vi "Dashboard Main.vi"() -> ()   [LabVIEW 2012]
uses:
  DIOOutput.ctl
  SensorsOutput.ctl
  <vilib>/event_ctls.llb/eventvkey.ctl
  <vilib>/Utility/config.llb/Read Key (String).vi
  <vilib>/Utility/config.llb/Read Key (I32).vi
  <vilib>/Utility/config.llb/Write Key (I32).vi
  <vilib>/Utility/config.llb/Write Key (String).vi
  <vilib>/Utility/config.llb/NI_LVConfig.lvlib
panel:
  out "LogFile 2":refnum<file>
  out "LogFile":refnum<file>
  in  "LogString":string
  out "Battery Value":dbl(slide) scale=0.0..14.0 scale format="%#_2e"
  out "Battery":sgl(graph)
  in  "Camera Settings":T1={"Frate Rate"=30, "Compression"=30, "Size"=1} {"Frate Rate" scale=1.0..30.0; "Size" items=["640x480", "320x240", "160x120"]}
  out "Mode":T2(ring)=enum."Auto Disabled"
  out "Camera IP":string
  out "JS1 Z":dbl(slide) scale=-1.0..1.0 scale format="%#_2e"
  out "JS2 Z":dbl(slide) scale=-1.0..1.0 scale format="%#_2e"
  out "Joystick 1":cluster{"X":dbl, "Y":dbl}[](graph)
  out "Joystick 2":cluster{"X":dbl, "Y":dbl}[](graph)
  out "JS Buttons 1":T3
  out "JS Buttons 2":T3
  out "MotorSlide4":dbl(slide) scale=-1.0..1.0 scale format="%#_2e"
  out "MotorSlide3":dbl(slide) scale=-1.0..1.0 scale format="%#_2e"
  out "MotorSlide2":dbl(slide) scale=-1.0..1.0 scale format="%#_2e"
  in  "MotorName3":string="Front Left"
  in  "MotorName4":string="Front Right"
  in  "MotorName1":string="Rear Left"
  in  "MotorName2":string="Rear Right"
  out "MotorChart4":dbl(graph)
  out "MotorChart3":dbl(graph)
  out "MotorChart2":dbl(graph)
  out "MotorSlide1":dbl(slide) scale=-1.0..1.0 scale format="%#_2e"
  out "MotorChart1":dbl(graph)
  out "Robot IP":string
  in  "Dashboard Tab":T4(tab)
  in  "Single Stick":bool
  in  "Shooter Scale":dbl(knob)=0.7000000000000001 min=0.1 max=1.0 step=0.1 scale=0.1..1.0 scale format="%#.1g"
  in  "Tank_Drive":bool
  out "DIO Template":T5
  out "Sensors":T6
  out "Target Info":T7(array[cluster])
  in  "Slider":dbl(slide) scale=0.0..100.0 scale format="%#_3g"
  in  "On/Off":bool caption="Solenoid"
  in  "Test Name":u16(ring) items=["Select the test to run...", "Example Test", "-------------------------------", "List of tests is built in robot code.", "Replace with your own automated tests."]
  in  "Test Tree":string(tree)
  in  "Motor":cluster{"Value":dbl, "Enable":bool} {"Value" scale=-1.0..1.0 scale format="%#_3g"}
  out "Progress":T8 {"Test Progress" scale=0.0..100.0}
  in  "Rev/Fwd":cluster{"Forward":bool, "Reverse":bool}
  in  "Ring":u16(ring) items=["Auto", "Fixed indoor", "Fixed outdoor 1", "Fixed outdoor 2", "Fixed fluorescent 1", "Fixed fluorescent 2", "Hold current"]
  in  "Listbox":i32(listbox)
  in  "Viewer":T9(tab)
  out "Mbps":dbl format="%#.1g"
  in  "Enable":bool
  in  "DB Camera Config":bool
  out "Mbps":bool
  out "fps":dbl format="%#.1g"
  out "Image Error Message":string="Timeout in Camera Communications"
  out "Camera Image":T10(plugin-control)
  out "Buttons 1":cluster{"1":bool, "2":bool, "3":bool}
  out "Kinect 1":cluster{"X":dbl, "Y":dbl, "Z":dbl} {"X" scale=1.0..-1.0; "Y" scale=1.0..-1.0; "Z" scale=1.0..-1.0}
  out "Buttons 2":cluster{"1":bool, "2":bool, "3":bool}
  out "Kinect 2":cluster{"X":dbl, "Y":dbl, "Z":dbl} {"X" scale=1.0..-1.0; "Y" scale=1.0..-1.0; "Z" scale=1.0..-1.0}
  out "Version":string
  out "Skeleton Picture":picture
  out "Players":i8
  out "Tree":string(tree)
  # "Drive & Motors"
  # "Robot IP:"
  # "Arcade Drive"
  # "Tank Drive"
  # "Double Stick"
  # "Single Stick"
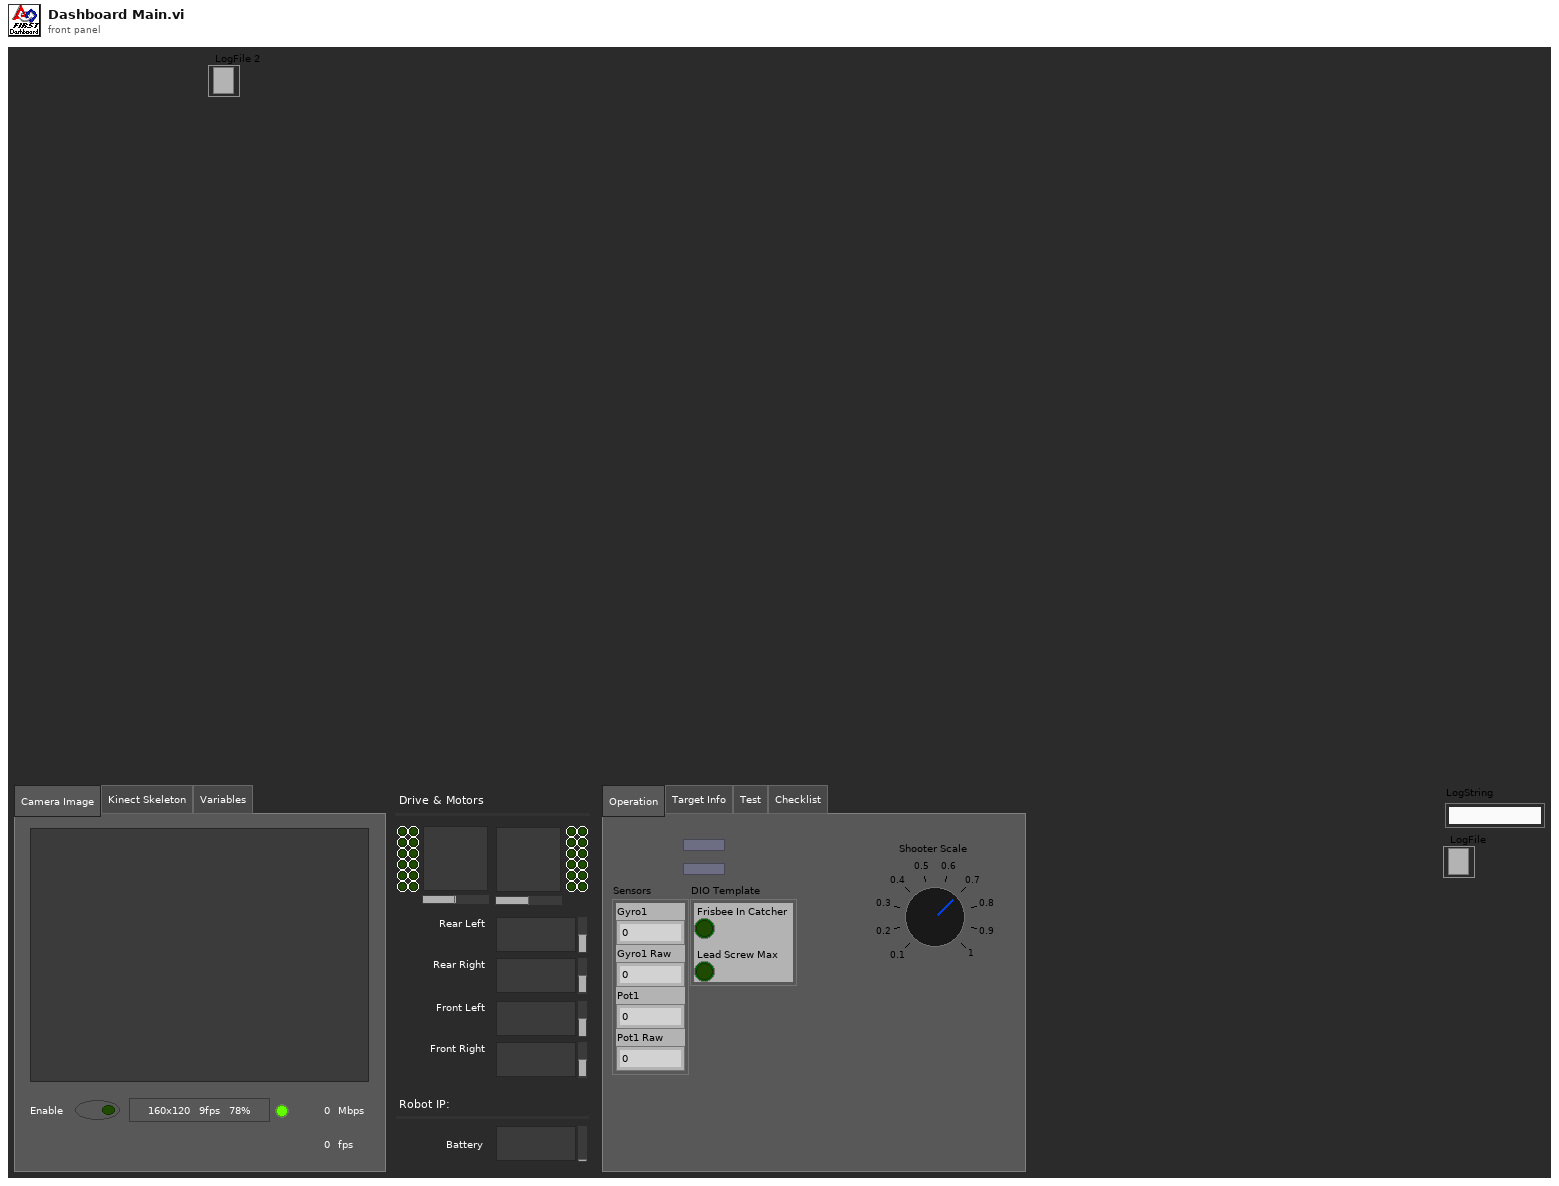
[diagram p1: front panel]
types:
  T1 = cluster{"Frate Rate":i32, "Compression":i32, "Size":u16}
  T2 = enum8{"Tele-Op Disabled", "Tele-Op Enabled", "Auto Disabled", "Auto Enabled", "Test Disabled", "Test Enabled", ""}
  T3 = cluster{bool, bool, bool, bool, bool, bool, bool, bool, bool, bool, bool, bool}
  T4 = enum32{"Operation", "Target Info", "Test", "Checklist"}
  T5 = typedef "DIOOutput.ctl" = cluster{"Frisbee In Catcher":bool, "Lead Screw Max":bool}
  T6 = typedef "SensorsOutput.ctl" = cluster{"Gyro1":dbl, "Gyro1 Raw":dbl, "Pot1":dbl, "Pot1 Raw":dbl}
  T7 = cluster{"Center Position":cluster{"X":dbl, "Y":dbl}, "Distance (ft)":dbl, "Center":bool}[]
  T8 = cluster{"Test Progress":u8, "Test Progress Text":string}
  T9 = enum32{"Camera Image", "Kinect Skeleton", "Variables"}
  T10 = typedef "IMAQ Image.ctl" = refnum<image>
  T11 = enum16{"open", "replace", "create", "open or create", "replace or create", "replace or create with confirmation"}
  T12 = typedef "Image Type" = u32
  T13 = typedef "LVBoundsTypeDef.ctl" = cluster{"Width":u32, "Height":u32}
  T14 = typedef "SkeletonTrackState.ctl" = enum32{"NotTracked", "PositionOnly", "Tracked"}
  T15 = cluster{"TrackingState":u8[], "Position":cluster{"x":sgl, "y":sgl, "z":sgl}, cluster{"x":sgl, "y":sgl, "z":sgl, sgl}[], "TrackState":T14}
  T16 = cluster{cluster{"ScaledToPercentRange":dbl, "ScaledToPercentRange":dbl, "ScaledToPercentRange":dbl}, cluster{bool, bool, bool}}[]
  T17 = cluster{cluster{"ScaledToPercentRange":dbl, "ScaledToPercentRange":dbl, "ScaledToPercentRange":dbl}, cluster{bool, bool, bool}}
  T18 = cluster{"ScaledToPercentRange":dbl, "ScaledToPercentRange":dbl, "ScaledToPercentRange":dbl}
  T19 = typedef "LVRectTypeDef.ctl" = cluster{"Left":i16, "Top":i16, "Right":i16, "Bottom":i16}
  T20 = cluster{"Competition mode":bool, "Robot Link":bool, "Autonomous":bool, "Enabled":bool, "E-Stop":bool, "Simulated":bool, "TestMode":bool, "Docked Window":bool}
  T21 = cluster{"Boolean Array[0]":bool, "Boolean Array[1]":bool, "Boolean Array[2]":bool, "Boolean Array[3]":bool, "Boolean Array[4]":bool, "Boolean Array[5]":bool, "Boolean Array[6]":bool, "Boolean Array[7]":bool, "Boolean Array[8]":bool, "Boolean Array[9]":bool, "Boolean Array[10]":bool, "Boolean Array[11]":bool}
  T22 = cluster{"Position":cluster{"X":dbl, "Y":dbl}, "Distance (ft)":dbl, "Center":bool}[]
  T23 = cluster{cluster{"Numeric":dbl, "Numeric":dbl}, "Numeric":dbl, bool}
  T24 = cluster{"Position":cluster{"Numeric":dbl, "Numeric":dbl}, "Numeric":dbl, "Center":bool}[]
  T25 = typedef "NI_LVConfig.lvlib/Config Data RefNum.ctl" = refnum<k1>
  T26 = typedef "LVDateTimeRec.ctl" = cluster{"fractional second":dbl, "second":i32, "minute":i32, "hour":i32, "day of month":i32, "month":i32, "year":i32, "day of week":i32, "day of year":i32, "DST":i32}
  T27 = typedef "eventvkey.ctl" = enum16{"ASCII", "Enter", "Return", "Shift", "Ctrl", "Alt", "Cmd", "Opt", "Caps", "NumLock", "Clear", "Break", "Up", "Down", "Left", "Right", "Insert", "Delete", "Home", "End", "PageUp", "PageDown", "Escape", "Help", "Pause", "ScrollLock", "F1", "F2", "F3", "F4", "F5", "F6", "F7", "F8", "F9", "F10", "F11", "F12", "F13", "F14", "F15", "F16", "F17", "F18", "F19", "F20", "F21", "F22", "F23", "F24", "Play", "VolumeUp", "VolumeDown", "Mute", "Two Byte Char"}
  T28 = cluster{"Numeric Array[0]":dbl, "Numeric Array[1]":dbl, "Numeric Array[2]":dbl, "Numeric Array[3]":dbl, "Numeric Array[4]":dbl, "Numeric Array[5]":dbl, "Numeric Array[6]":dbl, "Numeric Array[7]":dbl, "Numeric Array[8]":dbl}
  T29 = cluster{"Boolean Array[0]":bool, "Boolean Array[1]":bool, "Boolean Array[2]":bool, "Boolean Array[3]":bool, "Boolean Array[4]":bool, "Boolean Array[5]":bool, "Boolean Array[6]":bool, "Boolean Array[7]":bool, "Boolean Array[8]":bool}
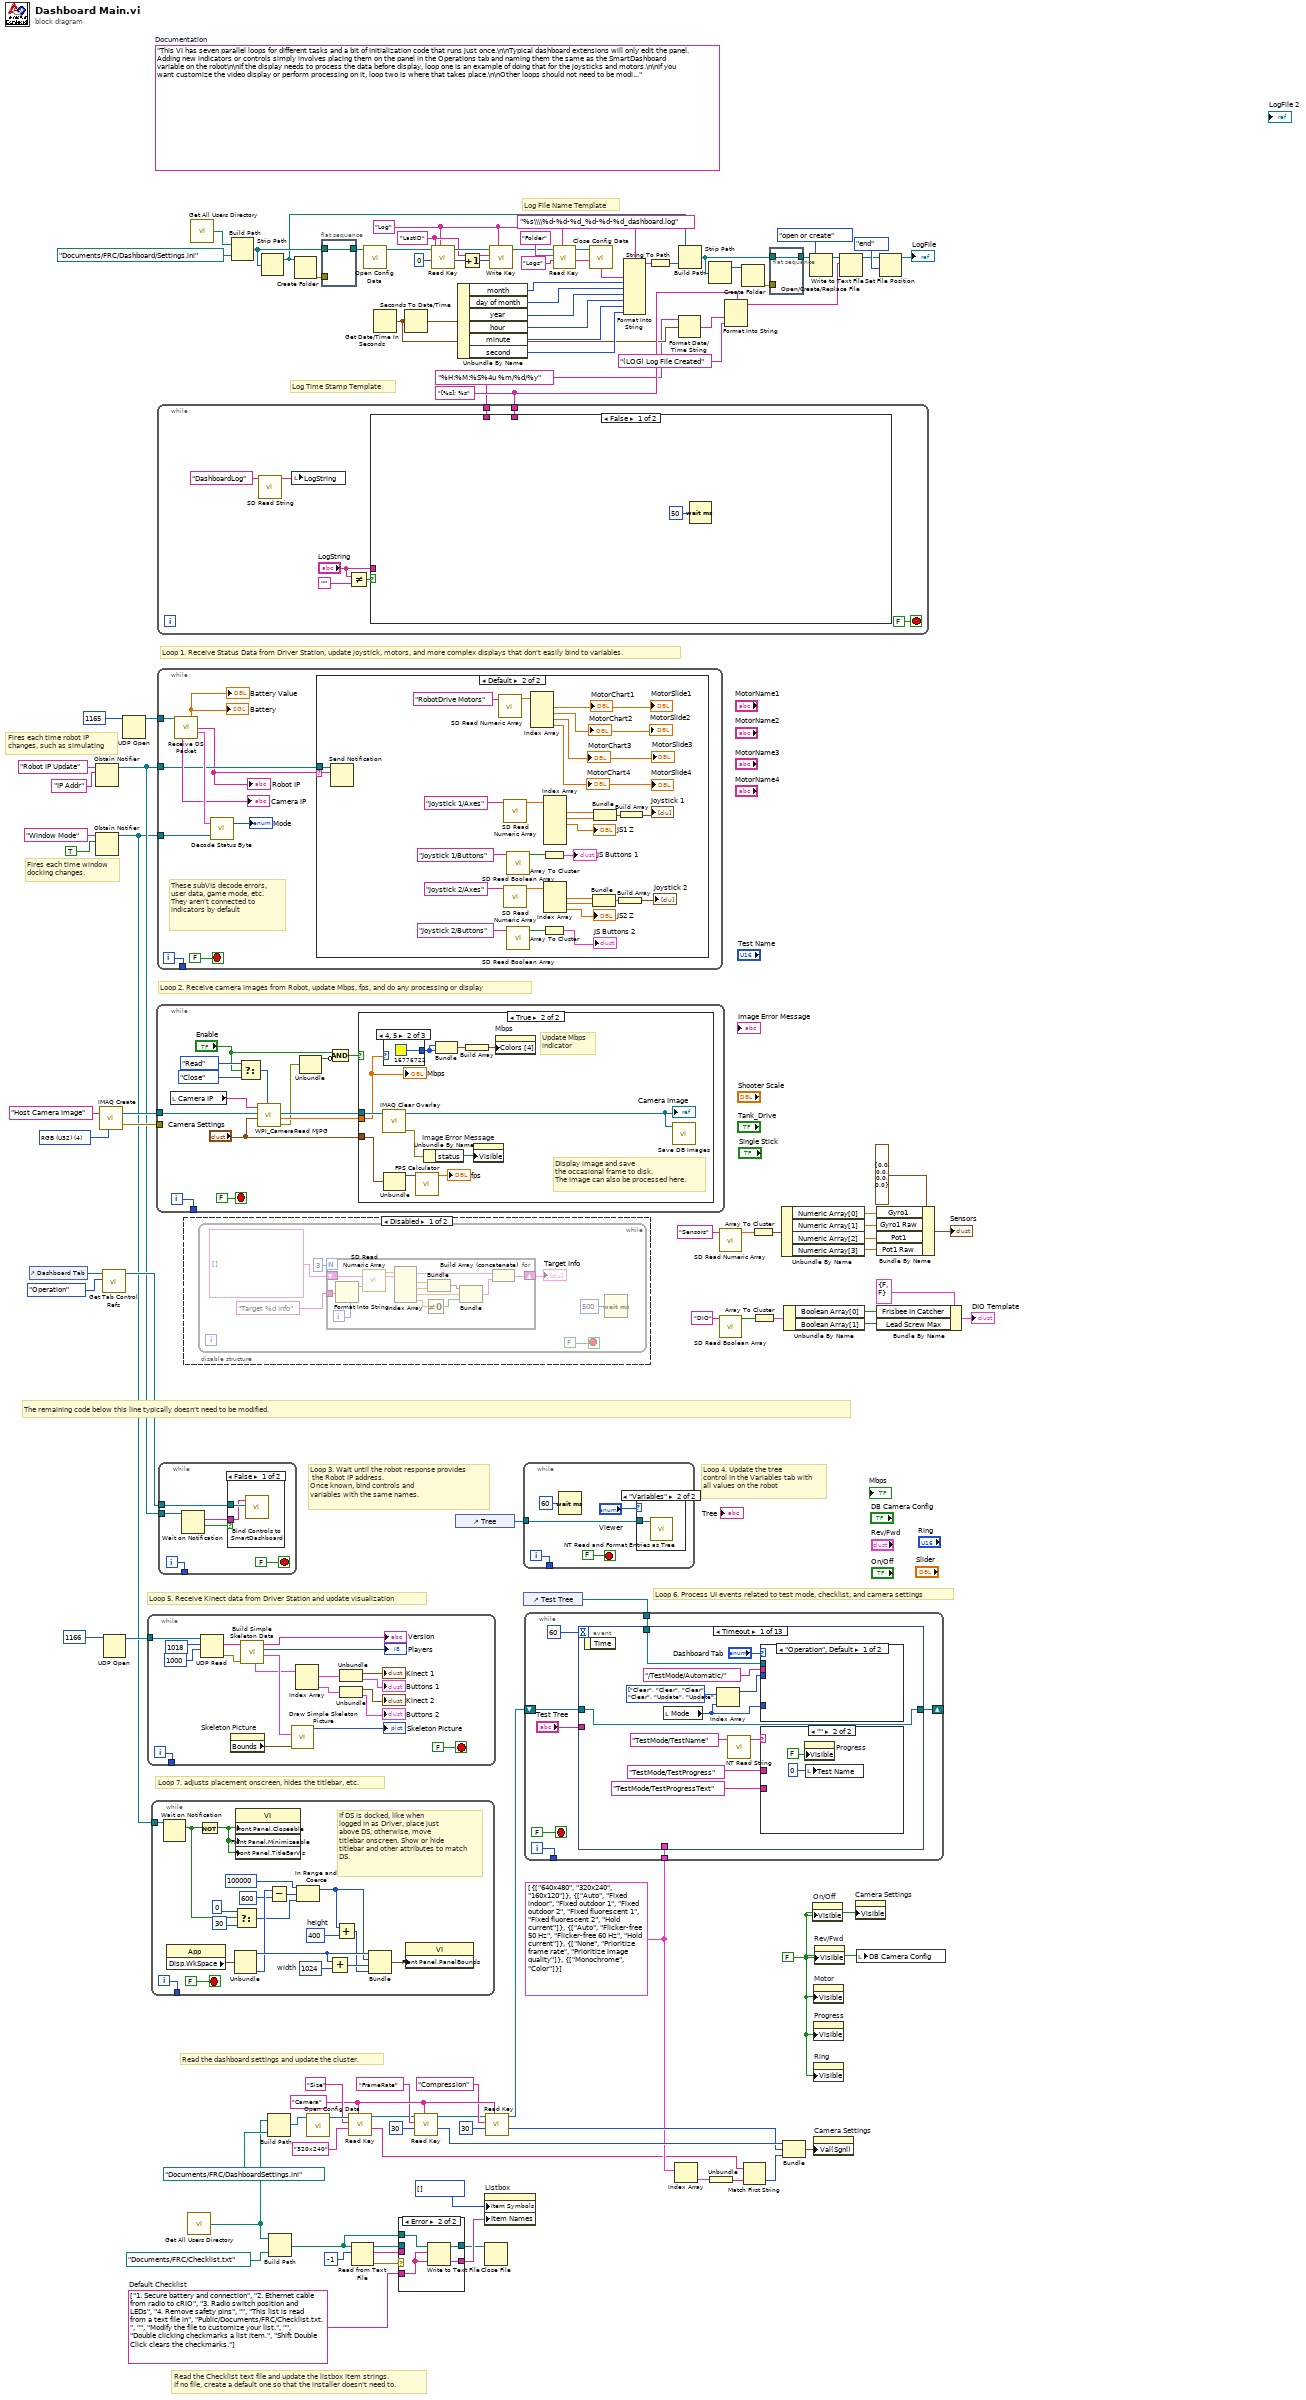
[diagram p0: block diagram]
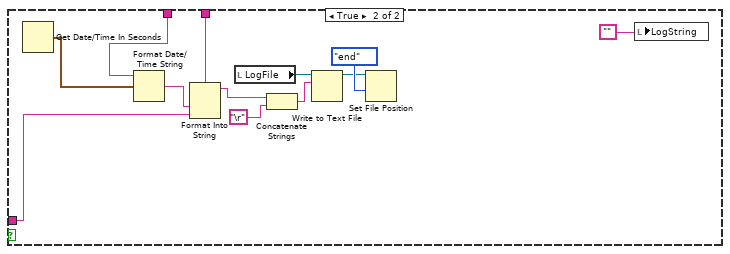
[diagram p2: hidden frame]
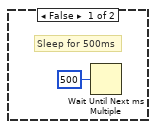
[diagram p5: hidden frame]
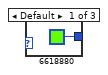
[diagram p6: hidden frame]
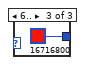
[diagram p7: hidden frame]
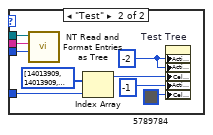
[diagram p9: hidden frame]
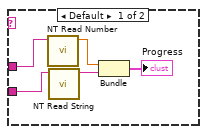
[diagram p10: hidden frame]
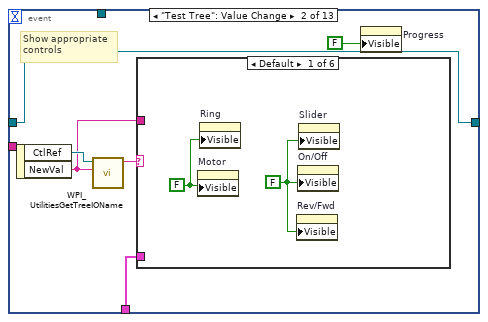
[diagram p11: hidden frame]
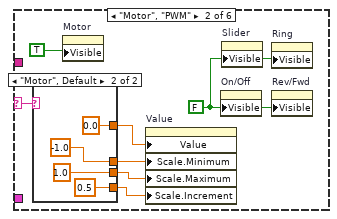
[diagram p12: hidden frame]
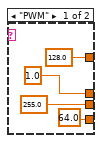
[diagram p13: hidden frame]
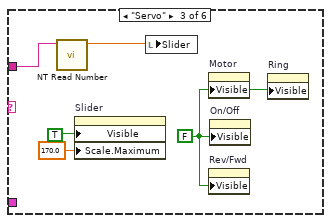
[diagram p14: hidden frame]
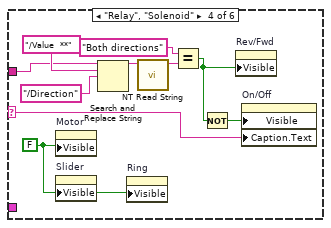
[diagram p15: hidden frame]
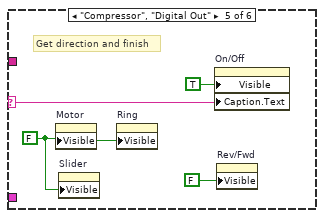
[diagram p16: hidden frame]
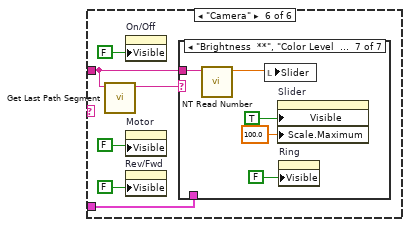
[diagram p17: hidden frame]
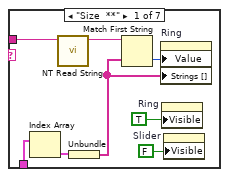
[diagram p18: hidden frame]
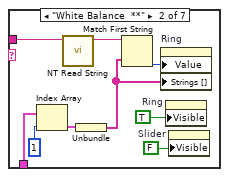
[diagram p19: hidden frame]
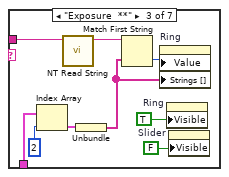
[diagram p20: hidden frame]
diagram:
  w17 = "%H:%M:%S%4u %m/%d/%y"
  w23 = "[%s]: %s"
  w50 = "LastID" ("key")
  w49 = "Log" ("section")
  w81 = "Camera"
  w73 = cluster{string[]}[] [{["640x480", "320x240", "160x120"]}, {["Auto", "Fixed indoor", "Fixed outdoor 1", "Fixed outdoor 2", "Fixed fluorescent 1", "Fixed fluorescent 2", "Hold current"]}, {["Auto", "Flicker-free 50 Hz", "Flicker-free 60 Hz", "Hold current"]}, {["None", "Prioritize frame rate", "Prioritize image quality"]}, {["Monochrome", "Color"]}]
  w88 = string[] ["1. Secure battery and connection", "2. Ethernet cable from radio to cRIO", "3. Radio switch position and LEDs", "4. Remove safety pins", "", "This list is read from a text file in", "Public/Documents/FRC/Checklist.txt.", "", "Modify the file to customize your list.", "", "Double clicking checkmarks a list item.", "Shift Double Click clears the checkmarks."]  # Default Checklist
  w86 = FALSE ("Visible")
  (unwired) "This VI has seven parallel loops for different tasks and a bit of initialization code that runs just once.\n\nTypical dashboard extensions will only edit the panel. Adding new indicators or controls simply involves placing them on the panel in the Operations tab and naming them the same as the SmartDashboard variable on the robot\n\nIf the display needs to process the data before display, loop one is an example of doing that for the joysticks and motors.\n\nIf you want customize the video display or perform processing on it, loop two is where that takes place.\n\nOther loops should not need to be modified. They are pretty standard, and document the task they perform."  # Documentation
  w109 = T12 4 items=["Grayscale (U8)", "Grayscale (I16)", "Grayscale (SGL)", "Complex (CSG)", "RGB (U32)", "HSL (U32)", "RGB (U64)"] ("Image Type")
  # "Log File Name Template"
  # "Log Time Stamp Template"
  # "Fires each time robot IP\nchanges, such as simulating"
  # "Fires each time window\ndocking changes."
  # "Read the Checklist text file and update the listbox item strings.\nIf no file, create a default one so that the installer doesn't need to."
  # "The remaining code below this line typically doesn't need to be modified."
  # "Loop 6. Process UI events related to test mode, checklist, and camera settings"
  # "Read the dashboard settings and update the cluster."
  # "Loop 4. Update the tree\ncontrol in the Variables tab with\nall values on the robot"
  # "Loop 3. Wait until the robot response provides\n the Robot IP address.\nOnce known, bind controls and\nvariables with the same names."
  # "Loop 5. Receive Kinect data from Driver Station and update visualization"
  # "Loop 7. adjusts placement onscreen, hides the titlebar, etc."
  # "Loop 1. Receive Status Data from Driver Station, update joystick, motors, and more complex displays that don't easily bind to variables."
  # "Loop 2. Receive camera images from Robot, update Mbps, fps, and do any processing or display"
  n1 = control-ref of="Dashboard Tab"() -> (w102:refnum<vi>)
  n2 = Obtain Notifier(name (unnamed)="Robot IP Update", notification data type="IP Addr" ("name (unnamed)")) -> (notifier out=w99:refnum<notifier>)  [unwired: 2 in, 2 out]
  n3 = Obtain Notifier(name (unnamed)="Window Mode", notification data type=TRUE) -> (notifier out=w92:refnum<notifier>)  [unwired: 2 in, 2 out]
  n4 = call "IMAQ Create"("Image Name"="Host Camera Image", "Image Type"=w109) -> ("New Image"=w107:T10, "error out"=w106:errorcluster)  [unwired: 2 in, 1 out]
  n5 = call <vilib>:"Get Tab Control Refs.vi"("Page Index"=enum32{"Operation", "Test"}."Operation" ("Dashboard Tab"), "TabControl in"=w102) -> ("ControlsOnPage"=w103:refnum<vi>[])  [unwired: 9 in]
  n6 = UDP Open(11:u16 1166 ("port")) -> (port=w104:refnum<k16>)  [unwired: 2 in, 4 out]
  n7 = UDP Open(11:u16 1165 ("port")) -> (port=w110:refnum<k16>)  [unwired: 2 in, 4 out]
  n8 = while {
    tunnel: w104 -> [w128]
    tunnel: [w113] -> _
    i -> [w113]
    stop <- FALSE stop-if-true
    n9 = UDP Read(connection ID=w128, max size (548)=1018 ("bytes to read"), timeout ms (25000)=1000) -> (data out=w122:string, error out=w112:errorcluster)  [unwired: 1 in, 3 out]
    n10 = property on="Skeleton Picture" class="Pict"() -> ("Bounds"=w124:T13)  [unwired: 2 in, 2 out]
    n11 = call "Build Simple Skeleton Data.vi"("error in (no error)"=w112, "data in"=w122) -> ("Skeleton Data"=w123:T15, "NumPlayers"=→"Players":i8, "Version String"=→"Version":string, "Simple Joystick Info"=w120:T16)  [unwired: 5 in, 1 out]
    n12 = call "Draw Simple Skeleton Picture.vi"("Bounds"=w124, "Simple Skeleton"=w123) -> ("new picture out"=→"Skeleton Picture":picture)  [unwired: 9 in]
    n13 = Index Array(array=w120) -> (element #1=w119:T17, element #2=w118:T17)  [unwired: 2 in]
    n14 = Unbundle(w119) -> (→"Kinect 1":T18, →"Buttons 1":cluster{bool, bool, bool})
    n15 = Unbundle(w118) -> (→"Kinect 2":T18, →"Buttons 2":cluster{bool, bool, bool})
  }
  n16 = while {
    tunnel: w92 -> [w149]
    tunnel: [w147] -> _
    i -> [w147]
    stop <- FALSE stop-if-true
    w139 = 1024  # width
    w142 = 400  # height
    # "If DS is docked, like when\nlogged in as Driver, place just\nabove DS, otherwise, move\ntitlebar onscreen. Show or hide\ntitlebar and other attributes to match\nDS."
    n17 = Wait on Notification(notifier=w149) -> (notification=w134:bool)  [unwired: 3 in, 3 out]
    n18 = property class="App"() -> ("Disp.WkSpace"=w145:T19)  [unwired: 2 in, 2 out]
    n19 = Not(x=w134) -> (.not. x?=w148:bool)
    n20 = Unbundle(w145) -> ("Left"=w143:i16, "Bottom"=w140:i16)  [unwired: 2 out]
    n21 = Select(t=0, s=w134, f=30) -> (s? t:f=w133:i32)
    n22 = property class="VI"("Front Panel.Closeable"=w148, "Front Panel.Minimizeable"=w148, "Front Panel.TitleBarVis"=w148) -> ()  [unwired: 2 in, 2 out]
    n23 = Subtract(x=w140, y=600) -> (x-y=w137:i32)
    n24 = In Range and Coerce(upper limit=100000, x=w137, lower limit=w133) -> (coerced(x)=w131:i32)  [unwired: 1 out]
    n25 = Add(x=w143, y=w139) -> (x+y=w144:i32)
    n26 = Add(x=w131, y=w142) -> (x+y=w141:i32)
    n27 = Bundle("Left"=w143, w131, w144, w141) -> (w146:cluster{"Left":i16, i32, i32, i32})  [unwired: 1 out]
    n28 = property class="VI"("Front Panel.PanelBounds"=w146) -> ()  [unwired: 2 in, 2 out]
  }
  n29 = while {
    tunnel: w107 -> [w160]
    tunnel: w106 -> [_]
    tunnel: [w163] -> _
    i -> [w163]
    stop <- FALSE stop-if-true
    n30 = local read "Camera IP"() -> (w162:string)
    n31 = Select(t=enum16{"Read", "Reopen", "Close"}."Read" ("Operation"), s="Enable", f=enum16{"Read", "Reopen", "Close"}."Close" ("Operation")) -> (s? t:f=w155:enum16{"Read", "Reopen", "Close"})
    n32 = call <vilib>:"WPI_CameraRead MJPG.vi"("Operation"=w155, "Camera Settings"="Camera Settings", "Image"=w160, "address"=w162) -> ("error out"=w154:errorcluster, "Bandwidth (kbps)"=w158:dbl, "Image Out"=w159:T10)  [unwired: 5 in]
    n33 = Unbundle(w154) -> ("status"=w152:bool)  [unwired: 2 out]
    n34 = Compound Arithmetic op=AND("Enable", invert w152) -> (w151:bool)
    n35 = case shown="True" w151 {
      tunnel: "Camera Settings" -> [_ w167]
      tunnel: w159 -> [_ w170]
      tunnel: w158 -> [_ w169]
      frame False {
        # "Sleep for 500ms"
        n36 = Wait Until Next ms Multiple(millisecond multiple=u32 500) -> ()  [unwired: 1 out]
      }
      frame True {
        # "Display image and save\nthe occasional frame to disk.\nThe image can also be processed here."
        # "Update Mbps\nindicator"
        n37 = call "IMAQ Clear Overlay"("Image"=w170) -> ("error out"=w175:errorcluster, "Image Out"=w174:T10)  [unwired: 2 in, 7 out]
        "Camera Image" <- w174
        n38 = case shown="4, 5" w169 {
          tunnel: [u32 6618880 ("Color Box") u32 16776722 ("Color Box") u32 16716800 ("Color Box")] -> w171
          frame Default {
          }
          frame 4, 5 {
          }
          frame 6.. {
          }
        }
        n39 = Unbundle(w167) -> ("Frate Rate"=w166:i32)  [unwired: 2 out]
        n40 = call "FPS Calculator.vi"("Average Count"=w166) -> ("fps"=→"fps":dbl)  [unwired: 10 in]
        n41 = Unbundle By Name(w175) -> ("status"=w176:bool)
        n42 = Bundle("Color Box"=w171, "Color Box"=w171) -> (w173:cluster{"Color Box":u32, "Color Box":u32})  [unwired: 1 out]
        n43 = Build Array(w173) -> (w172:cluster{"Color Box":u32, "Color Box":u32}[])
        n44 = property on="Image Error Message" class="Str"("Visible"=w176) -> ()  [unwired: 2 in, 2 out]
        n45 = property on="Mbps" class="Bool (strict)"("Colors [4]"=w172) -> ()  [unwired: 2 in, 2 out]
        n46 = call "Save DB Images.vi"("Image"=w174) -> ()  [unwired: 2 in, 1 out]
        "Mbps" <- w169
      }
    }
  }
  n47 = while {
    tunnel: w23 -> [w184]
    tunnel: w17 -> [w182]
    stop <- FALSE stop-if-true
    n48 = call <vilib>:"SD Read String.vi"("Name"="DashboardLog") -> ("String"=w180:string)  [unwired: 8 in, 2 out]
    n49 = local write "LogString"(w180) -> ()
    n50 = Not Equal?(x="LogString", y="") -> (x != y?=w186:bool)
    n51 = case shown="False" w186 {
      tunnel: "LogString" -> [_ w189]
      tunnel: w184 -> [_ w197]
      tunnel: w182 -> [_ w191]
      frame False {
        n52 = Wait (ms)(milliseconds to wait=u32 50) -> ()  [unwired: 1 out]
      }
      frame True {
        n53 = Get Date/Time In Seconds() -> (seconds since 1Jan1904=w192:timestamp)
        n54 = Format Date/Time String(time format string (%c)=w191, seconds (now)=w192) -> (date/time string=w190:string)  [unwired: 1 in]
        n55 = Format Into String(format string=w197, w190, w189) -> (resulting string=w194:string)  [unwired: 2 in, 1 out]
        n56 = local read "LogFile"() -> (w198:refnum<file>)
        n57 = Concatenate Strings(w194, "\r") -> (w195:string)
        n58 = Write to Text File(file (use dialog)=w198, text=w195) -> (refnum out=w199:refnum<file>)  [unwired: 2 in, 2 out]
        n59 = Set File Position(refnum=w199, from (0:start)=enum16{"start", "end", "current"}."end") -> ()  [unwired: 2 in, 2 out]
        n60 = local write "LogString"("") -> ()
      }
    }
  }
  n61 = while {
    tunnel: w110 -> [w208]
    tunnel: w99 -> [w202]
    tunnel: w92 -> [w206]
    tunnel: [w203] -> _
    i -> [w203]
    stop <- FALSE stop-if-true
    # "These subVIs decode errors, user data, game mode, etc.\nThey aren't connected to indicators by default"
    n62 = call "Receive DS Packet.vi"("Recv Socket"=w208) -> ("Battery"=→"Battery" →"Battery Value":sgl, "Robot IP Address"=w201:string, "Status"=w209:T20, "Camera IP Address"=→"Camera IP":string)  [unwired: 1 in, 10 out]
    "Robot IP" <- w201
    n63 = call "Decode Status Byte.vi"("Window Mode Notifier"=w206, "Status"=w209) -> ("Mode"=→"Mode":T2)  [unwired: 1 out]
    n64 = case shown="Default" w201 {
      selector: w201 -> [_ w211]
      tunnel: w202 -> [_ w212]
      frame "0.0.0.0" {
        # "Robot not responding, don't poll the variables"
      }
      frame Default {
        n65 = Send Notification(notification=w211, notifier=w212) -> ()  [unwired: 1 in, 2 out]
        n66 = call <vilib>:"SD Read Numeric Array.vi"("Name"="RobotDrive Motors") -> ("Numeric Array"=w235:dbl[])  [unwired: 8 in, 2 out]
        n67 = call <vilib>:"SD Read Numeric Array.vi"("Name"="Joystick 1/Axes") -> ("Numeric Array"=w228:dbl[])  [unwired: 8 in, 2 out]
        n68 = call <vilib>:"SD Read Numeric Array.vi"("Name"="Joystick 2/Axes") -> ("Numeric Array"=w222:dbl[])  [unwired: 8 in, 2 out]
        n69 = call <vilib>:"SD Read Boolean Array.vi"("Name"="Joystick 1/Buttons") -> ("Boolean Array"=w230:bool[])  [unwired: 8 in, 2 out]
        n70 = call <vilib>:"SD Read Boolean Array.vi"("Name"="Joystick 2/Buttons") -> ("Boolean Array"=w221:bool[])  [unwired: 8 in, 2 out]
        n71 = Index Array(array=w235) -> (element #1=→"MotorChart1" →"MotorSlide1":dbl, element #2=→"MotorSlide2" →"MotorChart2":dbl, element #3=→"MotorChart3" →"MotorSlide3":dbl, element #4=→"MotorChart4" →"MotorSlide4":dbl)  [unwired: 4 in]
        n72 = Array To Cluster(array=w230) -> (cluster=→"JS Buttons 1":T21)
        n73 = Array To Cluster(array=w221) -> (cluster=→"JS Buttons 2":T21)
        n74 = Index Array(array=w228) -> (element #1=w225:dbl, element #2=w226:dbl, element #3=→"JS1 Z":dbl)  [unwired: 6 in, 3 out]
        n75 = Index Array(array=w222) -> (element #1=w217:dbl, element #2=w216:dbl, element #3=→"JS2 Z":dbl)  [unwired: 3 in]
        n76 = Bundle("Numeric"=w217, "Numeric"=w216) -> (w218:cluster{"Numeric":dbl, "Numeric":dbl})  [unwired: 1 in]
        n77 = Bundle("Numeric"=w225, "Numeric"=w226) -> (w224:cluster{"Numeric":dbl, "Numeric":dbl})  [unwired: 1 in]
        n78 = Build Array(w218) -> (→"Joystick 2":cluster{"Numeric":dbl, "Numeric":dbl}[])
        n79 = Build Array(w224) -> (→"Joystick 1":cluster{"Numeric":dbl, "Numeric":dbl}[])
      }
    }
  }
  n80 = while {
    tunnel: w103 -> [w244]
    tunnel: w99 -> [w241]
    tunnel: [w239] -> _
    i -> [w239]
    stop <- FALSE stop-if-true
    n81 = Wait on Notification(notifier=w241) -> (notification=w240:string, timed out?=w242:bool)  [unwired: 3 in, 2 out]
    n82 = case shown="False" w242 {
      tunnel: w244 -> [w246 _]
      tunnel: w240 -> [w245 _]
      frame False {
        n83 = call <vilib>:"Bind Controls to SmartDashboard.vi"("Bound Control Refs"=w246, "Server IP Address"=w245) -> ()  [unwired: 10 in]
      }
      frame True {
      }
    }
  }
  n84 = disable-structure shown="Disabled" {
    frame Disabled {
      n85 = while {
        stop <- FALSE stop-if-true
        n86 = for {
          N: 3 -> [_]
          tunnel: "Target %d Info" ("format string") -> [w265]
          shift-right: [w253] -> w249
          shift-left: T22 [] -> [w254]
          i -> [w264]
          n87 = Format Into String(format string=w265, w264) -> (resulting string=w263:string)  [unwired: 2 in, 1 out]
          n88 = call <vilib>:"SD Read Numeric Array.vi"("Name"=w263) -> ("Numeric Array"=w262:dbl[])  [unwired: 8 in, 2 out]
          n89 = Index Array(array=w262) -> (element #1=w256:dbl, element #2=w257:dbl, element #3=w258:dbl, element #4=w261:dbl)  [unwired: 4 in]
          n90 = Not Equal To 0?(x=w261) -> (x != 0?=w260:bool)
          n91 = Bundle("Numeric"=w256, "Numeric"=w257) -> (w259:cluster{"Numeric":dbl, "Numeric":dbl})  [unwired: 1 in]
          n92 = Bundle(w259, "Numeric"=w258, w260) -> (w255:T23)  [unwired: 1 in]
          n93 = Build Array (concatenate)(w254, w255) -> (w253:T24)
        }
        "Target Info" <- w249
        n94 = Wait (ms)(milliseconds to wait=u32 500) -> ()  [unwired: 1 out]
      }
    }
    frame Enabled {
    }
  }
  n95 = call "Get All Users Directory.vi"() -> ("All User Path"=w46:path)
  n96 = call "Get All Users Directory.vi"() -> ("All User Path"=w38:path)
  n97 = Build Path(base path=w38, name or relative path=path "Documents/FRC/Dashboard/Settings.ini") -> (appended path=w43:path)
  n98 = Strip Path(path=w43) -> (stripped path=w35:path)  [unwired: 1 out]
  n99 = Build Path(base path=w46, name or relative path=path "Documents/FRC/DashboardSettings.ini") -> (appended path=w85:path)
  n100 = Build Path(base path=w46, name or relative path=path "Documents/FRC/Checklist.txt") -> (appended path=w89:path)
  n101 = Create Folder(path (use dialog)=w35) -> (error out=w44:errorcluster)  [unwired: 2 in, 2 out]
  n102 = call <vilib>:"Open Config Data.vi"("configuration file path"=w85) -> ("refnum"=w84:T25)  [unwired: 8 in, 2 out]
  n103 = flat-sequence {
    tunnel: w44 -> [_]
    tunnel: [w266] -> w42
    tunnel: w43 -> [w266]
    frame #0 {
    }
  }
  n104 = call-poly <vilib>:"Read Key.vi"("section"=w81, "default value"="320x240", "key"="Size", "refnum"=w84) -> ("value"=w71:string, "refnum out"=w66:T25)  [unwired: 2 in, 4 out]
  n105 = Read from Text File(file (use dialog)=w89, count=-1 ("timeout ms (25000)")) -> (refnum out=w68:refnum<file>, text=w90:string[], error out=w91:errorcluster)  [unwired: 2 in, 1 out]
  n106 = call <vilib>:"Open Config Data.vi"("configuration file path"=w42) -> ("refnum"=w59:T25)  [unwired: 8 in, 2 out]
  n107 = Get Date/Time In Seconds() -> (seconds since 1Jan1904=w18:timestamp)
  n108 = case shown="Error" w91 {
    tunnel: w90 -> [w268 _]
    tunnel: [w268 w270] -> w87
    tunnel: w88 -> [_ w270]
    tunnel: w89 -> [_ w271]
    tunnel: [w267 w269] -> w67
    tunnel: w68 -> [w267 _]
    frame No Error {
    }
    frame Error {
      n109 = Write to Text File(file (use dialog)=w271, text=w270) -> (refnum out=w269:refnum<file>)  [unwired: 2 in, 2 out]
    }
  }
  n110 = Seconds To Date/Time(time stamp (now)=w18) -> (date time rec=w33:T26)  [unwired: 1 in]
  n111 = call-poly <vilib>:"Read Key.vi"("section"=w81, "default value"=30, "key"="FrameRate", "refnum"=w66) -> ("value"=w76:i32, "refnum out"=w65:T25)  [unwired: 1 in, 5 out]
  n112 = call-poly <vilib>:"Read Key.vi"("section"=w49, "default value"=0, "key"=w50, "refnum"=w59) -> ("value"=w48:i32, "refnum out"=w52:T25)  [unwired: 4 in, 2 out]
  n113 = control-ref of="Tree"() -> (w62:refnum<vi>)
  n114 = Unbundle By Name(w33) -> ("month"=w22:i32, "day of month"=w21:i32, "year"=w27:i32, "hour"=w26:i32, "minute"=w25:i32, "second"=w24:i32)
  n115 = Increment(x=w48) -> (x+1=w45:i32)
  n116 = property on="Listbox" class="LstBox (strict)"("Item Symbols"=i32[] [], "Item Names"=w87) -> ()  [unwired: 2 in, 2 out]
  n117 = Close File(refnum=w67) -> ()  [unwired: 1 in, 2 out]
  n118 = call-poly <vilib>:"Read Key.vi"("section"=w81, "default value"=30, "key"="Compression", "refnum"=w65) -> ("value"=w75:i32, "refnum out"=w63:T25)  [unwired: 1 in, 5 out]
  n119 = call-poly <vilib>:"Write Key.vi"("section"=w49, "value"=w45, "key"=w50, "refnum"=w52) -> ("refnum out"=w51:T25)  [unwired: 5 in, 2 out]
  n120 = while {
    tunnel: [w273] -> _
    tunnel: w62 -> [w272]
    i -> [w273]
    stop <- FALSE stop-if-true
    n121 = Wait (ms)(milliseconds to wait=u32 60) -> ()  [unwired: 1 out]
    n122 = case shown="\"Variables\"" "Viewer" {
      tunnel: w272 -> [_ w277]
      frame Default {
      }
      frame "Variables" {
        n123 = call <vilib>:"NT Read and Format Entries as Tree.vi"("Tree Refnum"=w277) -> ()  [unwired: 9 in, 2 out]
      }
    }
  }
  n124 = control-ref of="Test Tree"() -> (w61:refnum<vi>)
  n125 = while {
    tunnel: w73 -> [w282]
    shift-right: [w281] -> _
    shift-left: w63 -> [w280]
    tunnel: [w279] -> _
    tunnel: w61 -> [w278]
    i -> [w279]
    stop <- FALSE stop-if-true
    n126 = event shown="[0] Timeout" {
      selector: _ -> [_ _ _ _ _ _ _ _ _ _ _ _ _]
      dyn-events: _ -> [_ _ _ _ _ _ _ _ _ _ _ _ _]
      timeout: u32 60 ("milliseconds to wait") -> [_ _ _ _ _ _ _ _ _ _ _ _ _]
      tunnel: w278 -> [w292 _ _ _ _ _ _ _ _ _ _ _ _]
      tunnel: "Test Tree" -> [_ _ _ _ _ _ _ _ w486 w494 w496 w500 w508]
      tunnel: w282 -> [_ w314 _ _ _ _ w450 w480 _ _ _ _ _]
      tunnel: [w286 w313 _ w416 w424 w436 w449 w473 w485 w492 w495 w499 w507] -> w281
      tunnel: w280 -> [w286 w313 _ w416 w424 w436 w448 w473 w485 w492 w495 w499 w507]
      event Timeout {
        w291 = enum16{"Update", "Clear"}[] [enum."Clear", enum."Clear", enum."Clear", enum."Clear", enum."Update", enum."Update", enum."Clear"] items=["Update", "Clear"]
        n127 = event-data() -> ()  [unwired: 1 in, 1 out]
        n128 = local read "Mode"() -> (w289:T2)
        n129 = Index Array(array=w291, index=w289) -> (element=w290:enum16{"Update", "Clear"})
        n130 = call <vilib>:"NT Read String.vi"("Name"="TestMode/TestName") -> ("String"=w295:string)  [unwired: 9 in, 1 out]
        n131 = case shown="\"Operation\", Default" "Dashboard Tab" {
          tunnel: w292 -> [_ w305]
          tunnel: "/TestMode/Automatic/" ("Name Pattern") -> [_ w304]
          tunnel: w290 -> [_ w303]
          tunnel: w289 -> [_ w301]
          frame "Operation", Default {
          }
          frame "Test" {
            w300 = -2 ("Active Item:Row Number")
            n132 = call <vilib>:"NT Read and Format Entries as Tree.vi"("Operation"=w303, "Name Pattern"=w304, "Tree Refnum"=w305) -> ()  [unwired: 7 in, 2 out]
            n133 = Index Array(array=u32[] [14013909, 14013909, 14013909, 14013909, 14013909, 16777215, 14013909], index=w301) -> (element=w299:u32)
            n134 = property on="Test Tree" class="Tree (strict)"("Active Item Row Number"=w300, "ActiveColNum"=w300, "CellBG"=w299, "Active Item Row Number"=-1 ("Active Item:Row Number"), "CellBG"=u32 5789784 ("Color Box")) -> ()  [unwired: 2 in, 2 out]
          }
        }
        n135 = case shown="\"\"" w295 {
          tunnel: "TestMode/TestProgress" ("Name") -> [w307 _]
          tunnel: "TestMode/TestProgressText" ("Name") -> [w306 _]
          frame Default {
            n136 = call <vilib>:"NT Read Number.vi"("Name"=w307) -> ("Numeric"=w308:dbl)  [unwired: 9 in, 1 out]
            n137 = call <vilib>:"NT Read String.vi"("Name"=w306) -> ("String"=w309:string)  [unwired: 9 in, 1 out]
            n138 = Bundle("Numeric"=w308, "String"=w309) -> (→"Progress":cluster{"Numeric":dbl, "String":string})  [unwired: 1 in]
          }
          frame "" {
            n139 = property on="Progress" class="Clust (strict)"("Visible"=FALSE) -> ()  [unwired: 2 in, 2 out]
            n140 = local write "Test Name"(u16 0) -> ()
          }
        }
      }
      event "Test Tree": Value Change {
        # "Show appropriate\ncontrols"
        n141 = event-data() -> ("CtlRef"=w317:refnum<vi>, "NewVal"=w315:string)  [unwired: 1 in]
        n142 = call <vilib>:"WPI_UtilitiesGetTreeIOName.vi"("NewVal"=w315, "TreeControl in"=w317) -> ("I/O Name"=w318:string)  [unwired: 9 in]
        n143 = case shown="Default" w318 {
          selector: w318 -> [_ w325 _ w343 w352 _]
          tunnel: w315 -> [_ _ w340 w342 _ w359]
          tunnel: w314 -> [_ _ _ _ _ w358]
          frame Default {
            w320 = FALSE ("Visible")
            w319 = FALSE ("Visible")
            n144 = property on="Motor" class="Clust (strict)"("Visible"=w319) -> ()  [unwired: 2 in, 2 out]
            n145 = property on="Ring" class="Ring (strict)"("Visible"=w319) -> ()  [unwired: 2 in, 2 out]
            n146 = property on="Rev/Fwd" class="Clust (strict)"("Visible"=w320) -> ()  [unwired: 2 in, 2 out]
            n147 = property on="On/Off" class="Bool (strict)"("Visible"=w320) -> ()  [unwired: 2 in, 2 out]
            n148 = property on="Slider" class="Slide (strict)"("Visible"=w320) -> ()  [unwired: 2 in, 2 out]
          }
          frame "Motor", "PWM" {
            w326 = FALSE ("Visible")
            n149 = case shown="\"Motor\", Default" w325 {
              tunnel: [1.0 ("Value") -1.0 ("Value")] -> w324
              tunnel: [255.0 ("Value") 1.0 ("Value")] -> w323
              tunnel: [128.0 ("Value") 0.0 ("Value")] -> w322
              tunnel: [64.0 ("Value") 0.5 ("Value")] -> w321
              frame "PWM" {
              }
              frame "Motor", Default {
              }
            }
            n150 = property on="Motor" class="Clust (strict)"("Visible"=TRUE) -> ()  [unwired: 2 in, 2 out]
            n151 = property on="Value" class="Slide (strict)"("Value"=w322, "Scale.Minimum"=w324, "Scale.Maximum"=w323, "Scale.Increment"=w321) -> ()  [unwired: 2 in, 2 out]
            n152 = property on="On/Off" class="Bool (strict)"("Visible"=w326) -> ()  [unwired: 2 in, 2 out]
            n153 = property on="Slider" class="Slide (strict)"("Visible"=w326) -> ()  [unwired: 2 in, 2 out]
            n154 = property on="Ring" class="Ring (strict)"("Visible"=w326) -> ()  [unwired: 2 in, 2 out]
            n155 = property on="Rev/Fwd" class="Clust (strict)"("Visible"=w326) -> ()  [unwired: 2 in, 2 out]
          }
          frame "Servo" {
            w338 = FALSE ("Visible")
            n156 = call <vilib>:"NT Read Number.vi"("Name"=w340) -> ("Numeric"=w339:dbl)  [unwired: 9 in, 1 out]
            n157 = property on="Slider" class="Slide (strict)"("Visible"=TRUE, "Scale.Maximum"=170.0 ("Scale.Range:Maximum")) -> ()  [unwired: 2 in, 2 out]
            n158 = local write "Slider"(w339) -> ()
            n159 = property on="Motor" class="Clust (strict)"("Visible"=w338) -> ()  [unwired: 2 in, 2 out]
            n160 = property on="Rev/Fwd" class="Clust (strict)"("Visible"=w338) -> ()  [unwired: 2 in, 2 out]
            n161 = property on="On/Off" class="Bool (strict)"("Visible"=w338) -> ()  [unwired: 2 in, 2 out]
            n162 = property on="Ring" class="Ring (strict)"("Visible"=w338) -> ()  [unwired: 2 in, 2 out]
          }
          frame "Relay", "Solenoid" {
            w341 = FALSE ("Visible")
            n163 = property on="Motor" class="Clust (strict)"("Visible"=w341) -> ()  [unwired: 2 in, 2 out]
            n164 = property on="Slider" class="Slide (strict)"("Visible"=w341) -> ()  [unwired: 2 in, 2 out]
            n165 = Search and Replace String(input string=w342, search string="/Value  **", replace string="/Direction") -> (result string=w348:string)  [unwired: 5 in, 3 out]
            n166 = property on="Ring" class="Ring (strict)"("Visible"=w341) -> ()  [unwired: 2 in, 2 out]
            n167 = call <vilib>:"NT Read String.vi"("Name"=w348) -> ("String"=w346:string)  [unwired: 9 in, 1 out]
            n168 = Equal?(x="Both directions", y=w346) -> (x = y?=w344:bool)
            n169 = Not(x=w344) -> (.not. x?=w345:bool)
            n170 = property on="Rev/Fwd" class="Clust (strict)"("Visible"=w344) -> ()  [unwired: 2 in, 2 out]
            n171 = property on="On/Off" class="Bool (strict)"("Visible"=w345, "Caption.Text"=w343) -> ()  [unwired: 2 in, 2 out]
          }
          frame "Compressor", "Digital Out" {
            w351 = FALSE ("Visible")
            # "Get direction and finish"
            n172 = property on="Motor" class="Clust (strict)"("Visible"=w351) -> ()  [unwired: 2 in, 2 out]
            n173 = property on="Slider" class="Slide (strict)"("Visible"=w351) -> ()  [unwired: 2 in, 2 out]
            n174 = property on="Ring" class="Ring (strict)"("Visible"=w351) -> ()  [unwired: 2 in, 2 out]
            n175 = property on="On/Off" class="Bool (strict)"("Visible"=TRUE, "Caption.Text"=w352) -> ()  [unwired: 2 in, 2 out]
            n176 = property on="Rev/Fwd" class="Clust (strict)"("Visible"=FALSE) -> ()  [unwired: 2 in, 2 out]
          }
          frame "Camera" {
            n177 = call <vilib>:"Get Last Path Segment.vi"("String in"=w359) -> ("String out"=w360:string)  [unwired: 10 in]
            n178 = property on="On/Off" class="Bool (strict)"("Visible"=FALSE) -> ()  [unwired: 2 in, 2 out]
            n179 = property on="Motor" class="Clust (strict)"("Visible"=FALSE) -> ()  [unwired: 2 in, 2 out]
            n180 = property on="Rev/Fwd" class="Clust (strict)"("Visible"=FALSE) -> ()  [unwired: 2 in, 2 out]
            n181 = case shown="\"Brightness  **\", \"Color Level  **\", \"Compression  **\", \"FPS  **\", \"Sharpness  **\"" w360 {
              tunnel: w359 -> [w366 w375 w384 w393 w402 _ w408]
              tunnel: w358 -> [w364 w372 w381 w390 w399 _ _]
              frame "Size  **" {
                n182 = Index Array(array=w364) -> (element=w363:cluster{string[]})  [unwired: 1 in]
                n183 = call <vilib>:"NT Read String.vi"("Name"=w366) -> ("String"=w365:string)  [unwired: 9 in, 1 out]
                n184 = Unbundle(w363) -> (w361:string[])
                n185 = Match First String(2:w361, 3:w365) -> (0:w362:i32)  [unwired: 1 out]
                n186 = property on="Ring" class="Ring (strict)"("Value"=w362, "Strings []"=w361) -> ()  [unwired: 2 in, 2 out]
                n187 = property on="Ring" class="Ring (strict)"("Visible"=TRUE) -> ()  [unwired: 2 in, 2 out]
                n188 = property on="Slider" class="Slide (strict)"("Visible"=FALSE) -> ()  [unwired: 2 in, 2 out]
              }
              frame "White Balance  **" {
                n189 = Index Array(array=w372, index=1) -> (element=w373:cluster{string[]})
                n190 = call <vilib>:"NT Read String.vi"("Name"=w375) -> ("String"=w374:string)  [unwired: 9 in, 1 out]
                n191 = Unbundle(w373) -> (w370:string[])
                n192 = Match First String(2:w370, 3:w374) -> (0:w369:i32)  [unwired: 1 out]
                n193 = property on="Ring" class="Ring (strict)"("Value"=w369, "Strings []"=w370) -> ()  [unwired: 2 in, 2 out]
                n194 = property on="Ring" class="Ring (strict)"("Visible"=TRUE) -> ()  [unwired: 2 in, 2 out]
                n195 = property on="Slider" class="Slide (strict)"("Visible"=FALSE) -> ()  [unwired: 2 in, 2 out]
              }
              frame "Exposure  **" {
                n196 = Index Array(array=w381, index=2) -> (element=w382:cluster{string[]})
                n197 = call <vilib>:"NT Read String.vi"("Name"=w384) -> ("String"=w383:string)  [unwired: 9 in, 1 out]
                n198 = Unbundle(w382) -> (w378:string[])
                n199 = Match First String(2:w378, 3:w383) -> (0:w379:i32)  [unwired: 1 out]
                n200 = property on="Ring" class="Ring (strict)"("Value"=w379, "Strings []"=w378) -> ()  [unwired: 2 in, 2 out]
                n201 = property on="Ring" class="Ring (strict)"("Visible"=TRUE) -> ()  [unwired: 2 in, 2 out]
                n202 = property on="Slider" class="Slide (strict)"("Visible"=FALSE) -> ()  [unwired: 2 in, 2 out]
              }
              frame "Exposure Priority  **" {
                n203 = Index Array(array=w390, index=3) -> (element=w391:cluster{string[]})
                n204 = call <vilib>:"NT Read String.vi"("Name"=w393) -> ("String"=w392:string)  [unwired: 9 in, 1 out]
                n205 = Unbundle(w391) -> (w387:string[])
                n206 = Match First String(2:w387, 3:w392) -> (0:w388:i32)  [unwired: 1 out]
                n207 = property on="Ring" class="Ring (strict)"("Value"=w388, "Strings []"=w387) -> ()  [unwired: 2 in, 2 out]
                n208 = property on="Ring" class="Ring (strict)"("Visible"=TRUE) -> ()  [unwired: 2 in, 2 out]
                n209 = property on="Slider" class="Slide (strict)"("Visible"=FALSE) -> ()  [unwired: 2 in, 2 out]
              }
              frame "Color Enable  **" {
                n210 = Index Array(array=w399, index=4) -> (element=w400:cluster{string[]})
                n211 = call <vilib>:"NT Read String.vi"("Name"=w402) -> ("String"=w401:string)  [unwired: 9 in, 1 out]
                n212 = Unbundle(w400) -> (w396:string[])
                n213 = Match First String(2:w396, 3:w401) -> (0:w397:i32)  [unwired: 1 out]
                n214 = property on="Ring" class="Ring (strict)"("Value"=w397, "Strings []"=w396) -> ()  [unwired: 2 in, 2 out]
                n215 = property on="Ring" class="Ring (strict)"("Visible"=TRUE) -> ()  [unwired: 2 in, 2 out]
                n216 = property on="Slider" class="Slide (strict)"("Visible"=FALSE) -> ()  [unwired: 2 in, 2 out]
              }
              frame Default {
                n217 = property on="Ring" class="Ring (strict)"("Visible"=FALSE) -> ()  [unwired: 2 in, 2 out]
                n218 = property on="Slider" class="Slide (strict)"("Visible"=FALSE) -> ()  [unwired: 2 in, 2 out]
              }
              frame "Brightness  **", "Color Level  **", "Compression  **", "FPS  **", "Sharpness  **" {
                n219 = call <vilib>:"NT Read Number.vi"("Name"=w408) -> ("Numeric"=w407:dbl)  [unwired: 9 in, 1 out]
                n220 = local write "Slider"(w407) -> ()
                n221 = property on="Slider" class="Slide (strict)"("Visible"=TRUE, "Scale.Maximum"=100.0 ("Scale.Range:Maximum")) -> ()  [unwired: 2 in, 2 out]
                n222 = property on="Ring" class="Ring (strict)"("Visible"=FALSE) -> ()  [unwired: 2 in, 2 out]
              }
            }
          }
        }
        n223 = property on="Progress" class="Clust (strict)"("Visible"=FALSE) -> ()  [unwired: 2 in, 2 out]
      }
      event "Test Name": Mouse Enter {
        # "Populate the ring with the list of tests"
        n224 = event-data() -> ()  [unwired: 1 in, 1 out]
        n225 = call <vilib>:"NT Read String Array.vi"("Name"="TestMode/TestList") -> ("String Array"=w415:string[])  [unwired: 9 in, 1 out]
        n226 = Build Array (concatenate)("Select the test to run...", w415) -> (w414:string[])
        n227 = property on="Test Name" class="Ring (strict)"("Strings []"=w414) -> ()  [unwired: 2 in, 2 out]
      }
      event "Test Name": Value Change {
        w417 = FALSE ("Visible")
        # "Tell the robot the test name to run"
        n228 = event-data() -> ("NewVal"=w421:u16)  [unwired: 1 in]
        n229 = property on="Test Name" class="Ring (strict)"() -> ("Strings []"=w422:string[])  [unwired: 2 in, 2 out]
        n230 = local write "Progress"(T8 {"Test Progress"=0, "Test Progress Text"=""} ("Progress")) -> ()
        n231 = Index Array(array=w422, index=w421) -> (element=w420:string)
        n232 = call <vilib>:"NT Write String.vi"("String"=w420, "Name"="TestMode/TestName") -> ()  [unwired: 9 in, 1 out]
        n233 = property on="Progress" class="Clust (strict)"("Visible"=TRUE) -> ()  [unwired: 2 in, 2 out]
        n234 = property on="Motor" class="Clust (strict)"("Visible"=w417) -> ()  [unwired: 2 in, 2 out]
        n235 = property on="Slider" class="Slide (strict)"("Visible"=w417) -> ()  [unwired: 2 in, 2 out]
        n236 = property on="On/Off" class="Bool (strict)"("Visible"=w417) -> ()  [unwired: 2 in, 2 out]
        n237 = property on="Rev/Fwd" class="Clust (strict)"("Visible"=w417) -> ()  [unwired: 2 in, 2 out]
        n238 = property on="Ring" class="Ring (strict)"("Visible"=w417) -> ()  [unwired: 2 in, 2 out]
      }
      event "Listbox": Double Click {
        n239 = event-data() -> ("PlatMods.Shift"=w425:bool, "Row"=w427:i32)  [unwired: 1 in]
        n240 = case shown="False" w425 {
          tunnel: w427 -> [w431 _]
          tunnel: 1 -> [w430 _]
          frame False {
            n241 = property on="Listbox" class="LstBox (strict)"() -> ("Item Symbols"=w429:i32[])  [unwired: 2 in, 2 out]
            n242 = Replace Array Subset(array=w429, new element=w430, index=w431) -> (w428:i32[])
            n243 = property on="Listbox" class="LstBox (strict)"("Item Symbols"=w428) -> ()  [unwired: 2 in, 2 out]
          }
          frame True {
            w432 = 0 ("Top Row")
            n244 = property on="Listbox" class="LstBox (strict)"() -> ("Number of Rows"=w434:u32)  [unwired: 2 in, 2 out]
            n245 = Initialize Array(0, w434) -> (w433:i32[])
            n246 = property on="Listbox" class="LstBox (strict)"("Top Row"=w432, "Value"=w432, "Item Symbols"=w433) -> ()  [unwired: 2 in, 2 out]
          }
        }
      }
      event "Listbox": Key Down {
        n247 = event-data() -> ("VKey"=w438:T27)  [unwired: 1 in]
        n248 = case shown="\"Left\", \"Right\"" w438 {
          selector: w438 -> [w443 _]
          tunnel: eventvkey."Left" ("VKey") -> [w441 _]
          frame "Left", "Right" {
            n249 = Equal?(x=w441, y=w443) -> (x = y?=w442:bool)
            n250 = Select(t=0, s=w442, f=1) -> (s? t:f=w444:i32)
            n251 = property on="Listbox" class="LstBox (strict)"() -> ("Item Symbols"=w447:i32[])  [unwired: 2 in, 2 out]
            n252 = Replace Array Subset(array=w447, new element=w444, index="Listbox") -> (w446:i32[])
            n253 = property on="Listbox" class="LstBox (strict)"("Item Symbols"=w446) -> ()  [unwired: 2 in, 2 out]
          }
          frame Default {
          }
        }
      }
      event "DB Camera Config": Value Change {
        n254 = event-data() -> ("NewVal"=w451:bool)  [unwired: 1 in]
        n255 = case shown="False" w451 {
          tunnel: w450 -> [w460 _]
          tunnel: [w453 w471] -> w449
          tunnel: w448 -> [w452 w471]
          frame False {
            w467 = "Camera"
            w470 = FALSE ("Visible")
            n256 = local read "Camera Settings"() -> (w459:T1)
            n257 = Index Array(array=w460) -> (element=w463:cluster{string[]})  [unwired: 1 in]
            n258 = Unbundle(w459) -> ("Frate Rate"=w458:i32, "Compression"=w457:i32, "Size"=w461:u16)
            n259 = Unbundle(w463) -> (w462:string[])
            n260 = Index Array(array=w462, index=w461) -> (element=w456:string)
            n261 = call-poly <vilib>:"Write Key.vi"("section"=w467, "value"=w456, "key"="Size", "refnum"=w452) -> ("refnum out"=w469:T25)  [unwired: 2 in, 5 out]
            n262 = call-poly <vilib>:"Write Key.vi"("section"=w467, "value"=w458, "key"="FrameRate", "refnum"=w469) -> ("refnum out"=w468:T25)  [unwired: 1 in, 6 out]
            n263 = property on="Camera Settings" class="Clust (strict)"("Visible"=w470) -> ()  [unwired: 2 in, 2 out]
            n264 = local write "DB Camera Config"(w470) -> ()
            n265 = call-poly <vilib>:"Write Key.vi"("section"=w467, "value"=w457, "key"="Compression", "refnum"=w468) -> ("refnum out"=w454:T25)  [unwired: 1 in, 6 out]
            n266 = call <vilib>:"Close Config Data.vi"("refnum"=w454) -> ("file path"=w455:path)  [unwired: 2 in, 8 out]
            n267 = call <vilib>:"Open Config Data.vi"("configuration file path"=w455) -> ("refnum"=w453:T25)  [unwired: 8 in, 2 out]
          }
          frame True {
            n268 = property on="Camera Settings" class="Clust (strict)"("Visible"=TRUE) -> ()  [unwired: 2 in, 2 out]
          }
        }
      }
      event "Camera Settings": Value Change {
        n269 = event-data() -> ("NewVal"=w484:T1)  [unwired: 1 in]
        n270 = Index Array(array=w480) -> (element=w479:cluster{string[]})  [unwired: 1 in]
        n271 = Unbundle(w484) -> ("Frate Rate"=w475:i32, "Compression"=w474:i32, "Size"=w477:u16)
        n272 = Unbundle(w479) -> (w478:string[])
        n273 = Index Array(array=w478, index=w477) -> (element=w476:string)
        n274 = Format Into String(format string="%s   %dfps   %d%%", w476, w475, w474) -> (resulting string=w481:string)  [unwired: 2 in, 1 out]
        n275 = Build Array(w481) -> (w482:string[])
        n276 = property on="DB Camera Config" class="Bool (strict)"("Strings [4]"=w482) -> ()  [unwired: 2 in, 2 out]
      }
      event "Motor.Enable": Value Change {
        n277 = event-data() -> ("NewVal"=w490:bool)  [unwired: 1 in]
        n278 = Unbundle("Motor") -> ("Value"=w489:dbl)  [unwired: 1 out]
        n279 = Select(t=w489, s=w490, f=0.0) -> (s? t:f=w487:dbl)
        n280 = call <vilib>:"NT Write Number.vi"("Numeric"=w487, "Name"=w486) -> ()  [unwired: 9 in, 1 out]
      }
      event "Slider": Value Change {
        n281 = event-data() -> ("NewVal"=w493:dbl)  [unwired: 1 in]
        n282 = call <vilib>:"NT Write Number.vi"("Numeric"=w493, "Name"=w494) -> ()  [unwired: 9 in, 1 out]
      }
      event "On/Off": Value Change {
        n283 = event-data() -> ("NewVal"=w498:bool)  [unwired: 1 in]
        n284 = Boolean To (0,1)(Boolean=w498) -> (0, 1=w497:i16)
        n285 = call <vilib>:"NT Write Number.vi"("Numeric"=w497, "Name"=w496) -> ()  [unwired: 9 in, 1 out]
      }
      event "Rev/Fwd": Value Change {
        n286 = event-data() -> ("NewVal.Forward"=w506:bool, "NewVal.Reverse"=w505:bool)  [unwired: 1 in]
        n287 = Boolean To (0,1)(Boolean=w506) -> (0, 1=w502:i16)
        n288 = Boolean To (0,1)(Boolean=w505) -> (0, 1=w504:i16)
        n289 = Negate(x=w504) -> (-x=w503:i16)
        n290 = Add(x=w502, y=w503) -> (x+y=w501:i16)
        n291 = call <vilib>:"NT Write Number.vi"("Numeric"=w501, "Name"=w500) -> ()  [unwired: 9 in, 1 out]
      }
      event "Ring": Value Change {
        n292 = event-data() -> ("NewVal"=w510:u16)  [unwired: 1 in]
        n293 = property on="Ring" class="Ring (strict)"() -> ("Strings []"=w511:string[])  [unwired: 2 in, 2 out]
        n294 = Index Array(array=w511, index=w510) -> (element=w509:string)
        n295 = call <vilib>:"NT Write String.vi"("String"=w509, "Name"=w508) -> ()  [unwired: 9 in, 1 out]
      }
    }
  }
  n296 = call-poly <vilib>:"Read Key.vi"("section"=w49, "default value"="Logs", "key"="Folder", "refnum"=w51) -> ("value"=w54:string, "refnum out"=w47:T25)  [unwired: 4 in, 2 out]
  n297 = call <vilib>:"Close Config Data.vi"("refnum"=w47) -> ()  [unwired: 9 in, 2 out]
  n298 = Format Into String(format string="%s\\\\%d-%d-%d_%d-%d-%d_dashboard.log", w54, w22, w21, w27, w26, w25, w24) -> (resulting string=w56:string)  [unwired: 2 in, 1 out]
  n299 = String To Path(string=w56) -> (path=w37:path)
  n300 = Index Array(array=w73) -> (element=w74:cluster{string[]})  [unwired: 1 in]
  n301 = Format Date/Time String(time format string (%c)=w17, seconds (now)=w18) -> (date/time string=w19:string)  [unwired: 1 in]
  n302 = Build Path(base path=w35, name or relative path=w37) -> (appended path=w39:path)
  n303 = Strip Path(path=w39) -> (stripped path=w41:path)  [unwired: 1 out]
  n304 = Unbundle(w74) -> (w72:string[])
  n305 = call <vilib>:"SD Read Numeric Array.vi"("Name"="Sensors") -> ("Numeric Array"=w15:dbl[])  [unwired: 8 in, 2 out]
  n306 = call <vilib>:"SD Read Boolean Array.vi"("Name"="DIO") -> ("Boolean Array"=w9:bool[])  [unwired: 8 in, 2 out]
  n307 = Format Into String(format string=w23, w19, "(LOG) Log File Created" ("input 7")) -> (resulting string=w30:string)  [unwired: 2 in, 1 out]
  n308 = Create Folder(path (use dialog)=w41) -> (error out=w40:errorcluster)  [unwired: 2 in, 2 out]
  n309 = Match First String(2:w72, 3:w71) -> (0:w70:i32)  [unwired: 1 out]
  n310 = Array To Cluster(array=w15) -> (cluster=w14:T28)
  n311 = Array To Cluster(array=w9) -> (cluster=w8:T29)
  n312 = flat-sequence {
    tunnel: w40 -> [_]
    tunnel: [w512] -> w36
    tunnel: w39 -> [w512]
    frame #0 {
    }
  }
  n313 = Unbundle By Name(w14) -> ("Numeric Array[0]"=w13:dbl, "Numeric Array[1]"=w12:dbl, "Numeric Array[2]"=w11:dbl, "Numeric Array[3]"=w10:dbl)
  n314 = Bundle("value"=w76, "value"=w75, "index"=w70) -> (w64:cluster{"value":i32, "value":i32, "index":i32})  [unwired: 1 out]
  n315 = Unbundle By Name(w8) -> ("Boolean Array[0]"=w7:bool, "Boolean Array[1]"=w5:bool)
  n316 = Open/Create/Replace File(file path (use dialog)=w36, operation (0:open)=T11."open or create") -> (refnum out=w29:refnum<file>)  [unwired: 4 in, 2 out]
  n317 = property on="On/Off" class="Bool (strict)"("Visible"=w86) -> ()  [unwired: 2 in, 2 out]
  n318 = property on="Motor" class="Clust (strict)"("Visible"=w86) -> ()  [unwired: 2 in, 2 out]
  n319 = property on="Progress" class="Clust (strict)"("Visible"=w86) -> ()  [unwired: 2 in, 2 out]
  n320 = property on="Ring" class="Ring (strict)"("Visible"=w86) -> ()  [unwired: 2 in, 2 out]
  n321 = property on="Camera Settings" class="Clust (strict)"("Val(Sgnl)"=w64) -> ()  [unwired: 2 in, 2 out]
  n322 = property on="Rev/Fwd" class="Clust (strict)"("Visible"=w86) -> ()  [unwired: 2 in, 2 out]
  n323 = Write to Text File(file (use dialog)=w29, text=w30) -> (refnum out=w31:refnum<file>)  [unwired: 2 in, 2 out]
  n324 = property on="Camera Settings" class="Clust (strict)"("Visible"=w86) -> ()  [unwired: 2 in, 2 out]
  n325 = local write "DB Camera Config"(w86) -> ()
  n326 = Bundle By Name(cluster=T6 {"Gyro1"=0.0, "Gyro1 Raw"=0.0, "Pot1"=0.0, "Pot1 Raw"=0.0} ("Sensors Template"), "Gyro1"=w13, "Gyro1 Raw"=w12, "Pot1"=w11, "Pot1 Raw"=w10) -> (→"Sensors":T6)
  n327 = Bundle By Name(cluster=T5 {"Frisbee In Catcher"=FALSE, "Lead Screw Max"=FALSE} ("DIO Template"), "Frisbee In Catcher"=w7, "Lead Screw Max"=w5) -> (→"DIO Template":T5)
  n328 = Set File Position(refnum=w31, from (0:start)=enum16{"start", "end", "current"}."end") -> (refnum out=→"LogFile":refnum<file>)  [unwired: 2 in, 1 out]
